vi "Generate write queue item.vi"(8 "error in (no error)":errorcluster, 11 "IAbort_rename in":refnum<class "IAbort.lvclass">) -> (0 "error out":errorcluster, 2 "Write queue item":T1, 3 "IAbort_rename out":refnum<class "IAbort.lvclass">)   [LabVIEW 2020, in "wamplv.lvlib" / "IAbort.lvclass"]
uses:
  IAbort.lvclass
  TypeDefs/Transport type.ctl
  wamplv.lvlib
  WAMP Client/Private/TypeDef/Write queue item.ctl
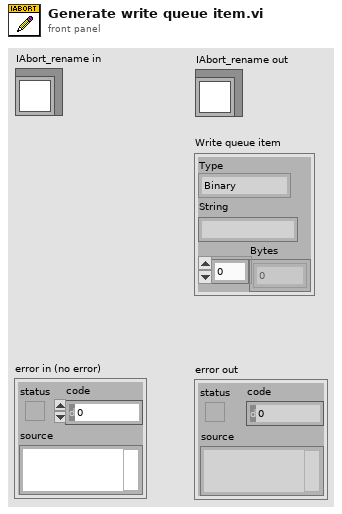
[diagram p1: front panel]
types:
  T1 = typedef "wamplv.lvlib/Write queue item.ctl" = cluster{"Type":T2, "String":string, "Bytes":u8[]}
  T2 = typedef "wamplv.lvlib/Transport type.ctl" = enum16{"Binary", "Text"}
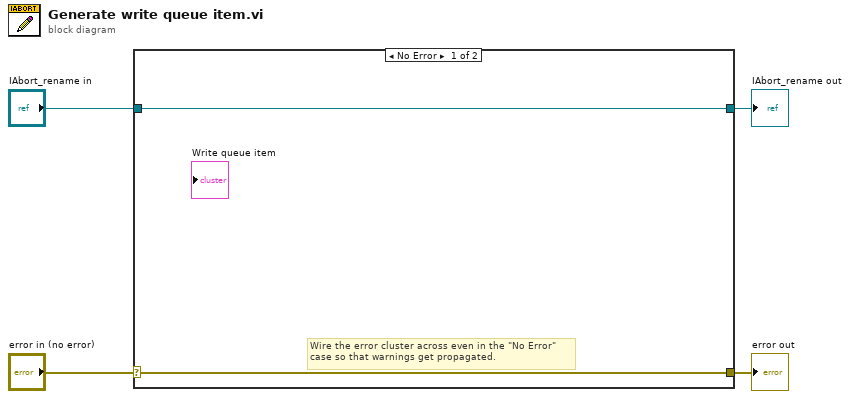
[diagram p0: block diagram]
diagram:
  n1 = case shown="No Error" "error in (no error)" {
    selector: "error in (no error)" -> [w5 w8]
    tunnel: [w5 w8] -> w3
    tunnel: [w6 w7] -> w1
    tunnel: "IAbort_rename in" -> [w6 w7]
    frame No Error {
      # "Wire the error cluster across even in the \"No Error\"\ncase so that warnings get propagated."
    }
    frame Error {
    }
  }
  "error out" <- w3
  "IAbort_rename out" <- w1
